vi "history-par.vi"(0 "device_id":string, 1 "sensor":string, 2 "limit":i32, 3 "base url":string) -> (7 "String":string, 8 "history":cluster{i32, "value":dbl}[](array[cluster]))   [LabVIEW 2026]
uses:
  <vilib>/addons/_JKI.lib/REST Client/classes/REST Client/REST Client.lvclass
panel:
  out "error out":errorcluster
  in  "error in (no error)":errorcluster
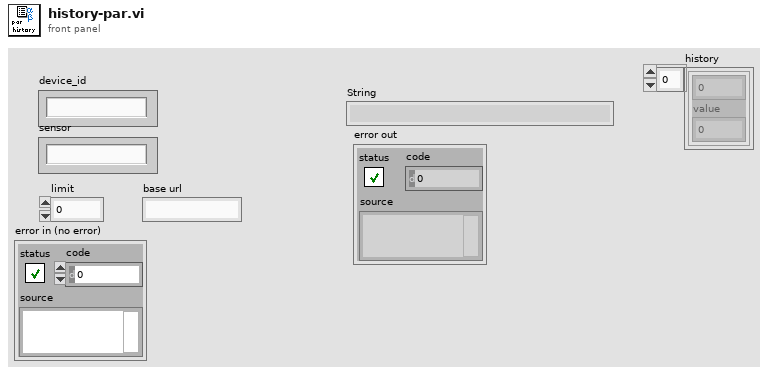
[diagram p1: front panel]
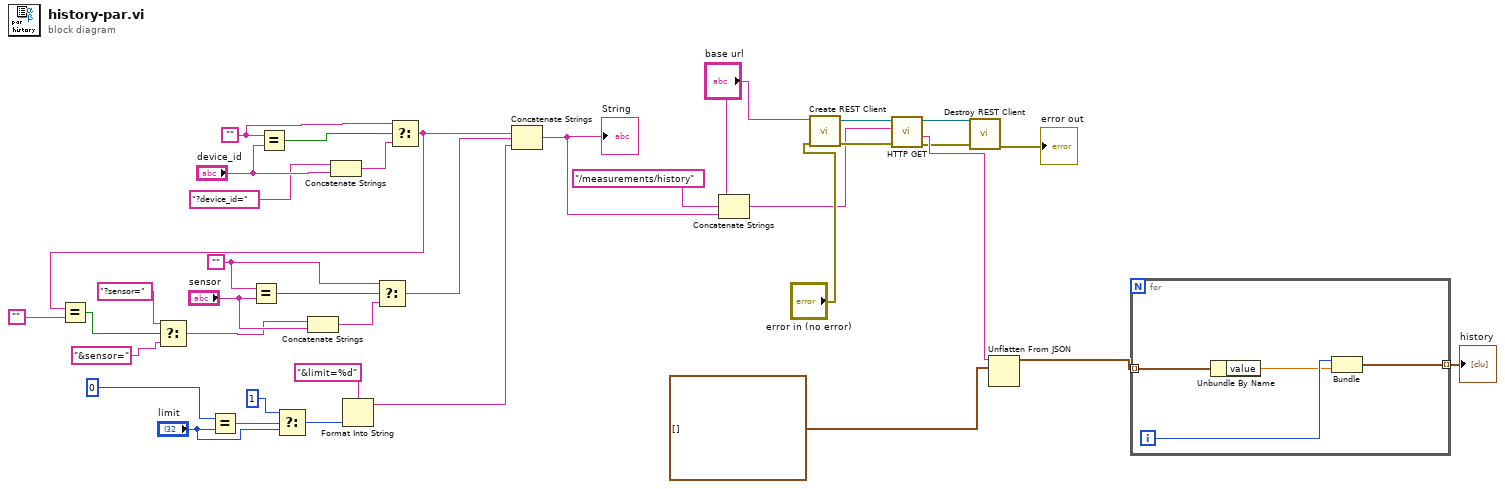
[diagram p0: block diagram]
diagram:
  w31 = ""
  w34 = ""
  n1 = Equal?(x=0, y="limit") -> (x = y?=w27:bool)
  n2 = Equal?(x=w31, y="sensor") -> (x = y?=w32:bool)
  n3 = Equal?(x=w34, y="device_id") -> (x = y?=w33:bool)
  n4 = Select(t=1 ("x"), s=w27, f="limit") -> (s? t:f=w24:i32)
  n5 = Concatenate Strings("?device_id=" ("string"), "device_id") -> (w37:string)
  n6 = Format Into String(format string="&limit=%d", w24) -> (resulting string=w21:string)  [unwired: 2 in, 1 out]
  n7 = Select(t=w34, s=w33, f=w37) -> (s? t:f=w20:string)
  n8 = Equal?(x=w20, y="") -> (x = y?=w18:bool)
  n9 = Select(t="?sensor=" ("string"), s=w18, f="&sensor=" ("string")) -> (s? t:f=w15:string)
  n10 = Concatenate Strings(w15, "sensor") -> (w29:string)
  n11 = Select(t=w31, s=w32, f=w29) -> (s? t:f=w22:string)
  n12 = Concatenate Strings(w20, w22, w21) -> (w13:string)
  "String" <- w13
  n13 = Concatenate Strings("base url", "/measurements/history" ("string"), w13) -> (w2:string)
  n14 = call <vilib>:"Create REST Client.vi"("error in (no error)"="error in (no error)", "Base URL"="base url") -> ("error out"=w8:errorcluster, "REST Client out"=w12:refnum<class "REST Client.lvclass">)  [unwired: 8 in]
  n15 = call-dynamic "HTTP GET.vi"("error in (no error)"=w8, "Path"=w2, "REST Client in"=w12) -> ("error out"=w7:errorcluster, "Response body"=w10:string, "REST Client out"=w11:refnum<class "REST Client.lvclass">)  [unwired: 3 in, 3 out]
  n16 = call-dynamic "Destroy REST Client.vi"("error in (no error)"=w7, "REST Client in"=w11) -> ("error out"=→"error out":errorcluster)  [unwired: 9 in]
  n17 = Unflatten From JSON(JSON string=w10, type and defaults=cluster{"value":dbl}[] []) -> (value=w4:cluster{"value":dbl}[])  [unwired: 5 in, 1 out]
  n18 = for {
    tunnel: w4 -> [w41] mode=indexing
    tunnel: [w38] -> w1 mode=indexing
    i -> [w40]
    n19 = Unbundle By Name(w41) -> ("value"=w39:dbl)
    n20 = Bundle(w40, "value"=w39) -> (w38:cluster{i32, "value":dbl})  [unwired: 1 in]
  }
  "history" <- w1
